vi "LBCB Conversion Unit Test.vi"() -> ()   [LabVIEW 2009]
uses:
  lib/Data Access Objects/Metadata/Actuator Point.ctl
  lib/Data Access Objects/Metadata/Cartesian Point.ctl
  lib/Data Access Objects/Metadata/Cartesian Force Vector.ctl
  lib/Data Access Objects/Metadata/LBCB Number.ctl
  lib/Data Access Objects/Metadata/LBCB Settings.ctl
  lib/Data Access Objects/Metadata/LBCB Size.ctl
  lib/Data Access Objects/Metadata/LBCB Type.ctl
  lib/Data Access Objects/Metadata/LBCB Location.ctl
  lib/Data Access Objects/Metadata/LBCB Position.ctl
  lib/Data Access Objects/Metadata/Persistant DAO Actions.ctl
  lib/Control Loop/LBCB_Conversions_Actions.ctl
panel:
  out "Filename Out":path
  in  "LBCB Position":T1={"Motion Center"=[0.0, 0.0, 0.0], "Transformation Matrix"=[[1.0, 0.0, 0.0, 0.0, 0.0, 0.0], [0.0, 1.0, 0.0, 0.0, 0.0, 0.0], [0.0, 0.0, 1.0, 0.0, 0.0, 0.0], [0.0, 0.0, 0.0, 1.0, 0.0, 0.0], [0.0, 0.0, 0.0, 0.0, 1.0, 0.0], [0.0, 0.0, 0.0, 0.0, 0.0, 1.0]]} {"Transformation Matrix" format="%#_10e"; "Motion Center" format="%#_10g"}
  in  "Save":bool
  in  "Load":bool
  in  "OM  Location":T2
  in  "Calculate":bool
  in  "LBCB Setting":T3
  in  "LBCB Number":T6
  in  "Stop":bool
  out "Forces":T7
  out "Displacements":T8
  in  "Forces Kips":T9
  in  "Displacements Inches":T9
  # "Y"
  # "(inch)"
  # "XLBCB CMD = T-1*XLBCB OM"
  # "Z"
  # "(inch)"
  # "XOM DISP = T*XLBCB DISP"
  # "(inch)"
  # "Dx"
  # "Dy"
  # "Dz"
  # "Rx"
  # "Ry"
  # "Rz"
  # "Dx"
  # "Dy"
  # "Dz"
  # "Rx"
  # "Ry"
  # "Rz"
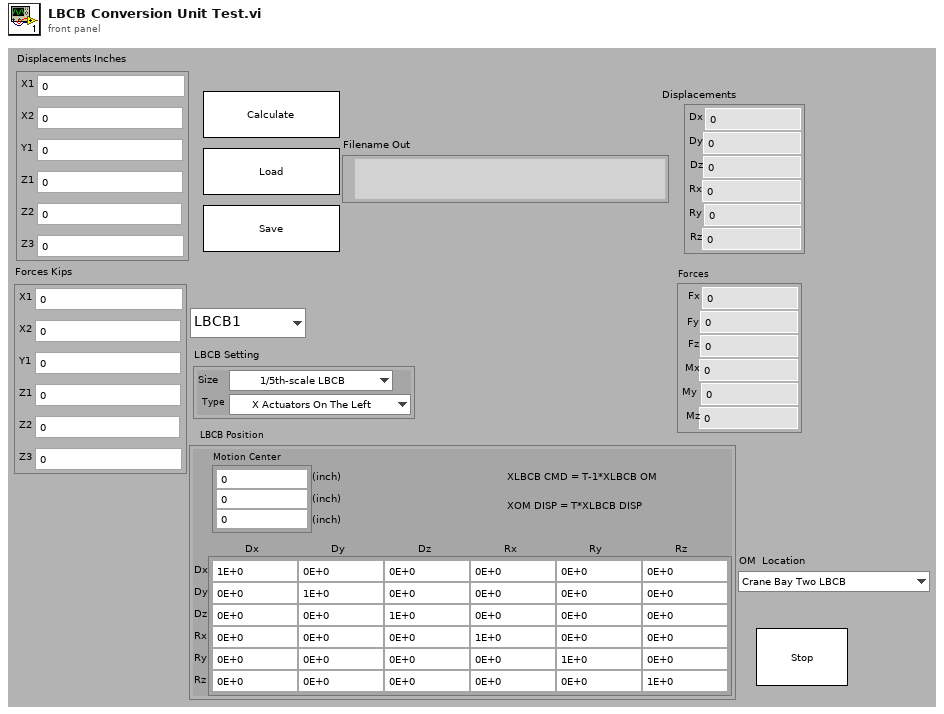
[diagram p1: front panel]
types:
  T1 = typedef "LBCB Position.ctl" = cluster{"Motion Center":dbl[], "Transformation Matrix":dbl[][]}
  T2 = typedef "LBCB Location.ctl" = enum16{"Crane Bay Two LBCB", "Crane Bay One LBCB", "5th Scale Two LBCB", "5th Scale One LBCB", "Portable LBCB"}
  T3 = typedef "LBCB Settings.ctl" = cluster{"Size":T4, "Type":T5}
  T4 = typedef "LBCB Size.ctl" = enum16{"1/5th-scale LBCB", "Full-scale LBCB", "Portable LBCB"}
  T5 = typedef "LBCB Type.ctl" = enum16{"X Actuators On The Left", "X Actuators On The Right"}
  T6 = typedef "LBCB Number.ctl" = enum16{"LBCB1", "LBCB2"}
  T7 = typedef "Cartesian Force Vector.ctl" = cluster{"Fx":dbl, "Fy":dbl, "Fz":dbl, "Mx":dbl, "My":dbl, "Mz":dbl}
  T8 = typedef "Cartesian Point.ctl" = cluster{"Dx":dbl, "Dy":dbl, "Dz":dbl, "Rx":dbl, "Ry":dbl, "Rz":dbl}
  T9 = typedef "Actuator Point.ctl" = cluster{"X1":dbl, "X2":dbl, "Y1":dbl, "Z1":dbl, "Z2":dbl, "Z3":dbl}
  T10 = typedef "Persistant DAO Actions.ctl" = enum16{"Init", "Get", "Set", "Load", "Save"}
  T11 = typedef "LBCB_Conversions_Actions.ctl" = enum16{"A2C", "C2A", "Set Log Filename", "Init"}
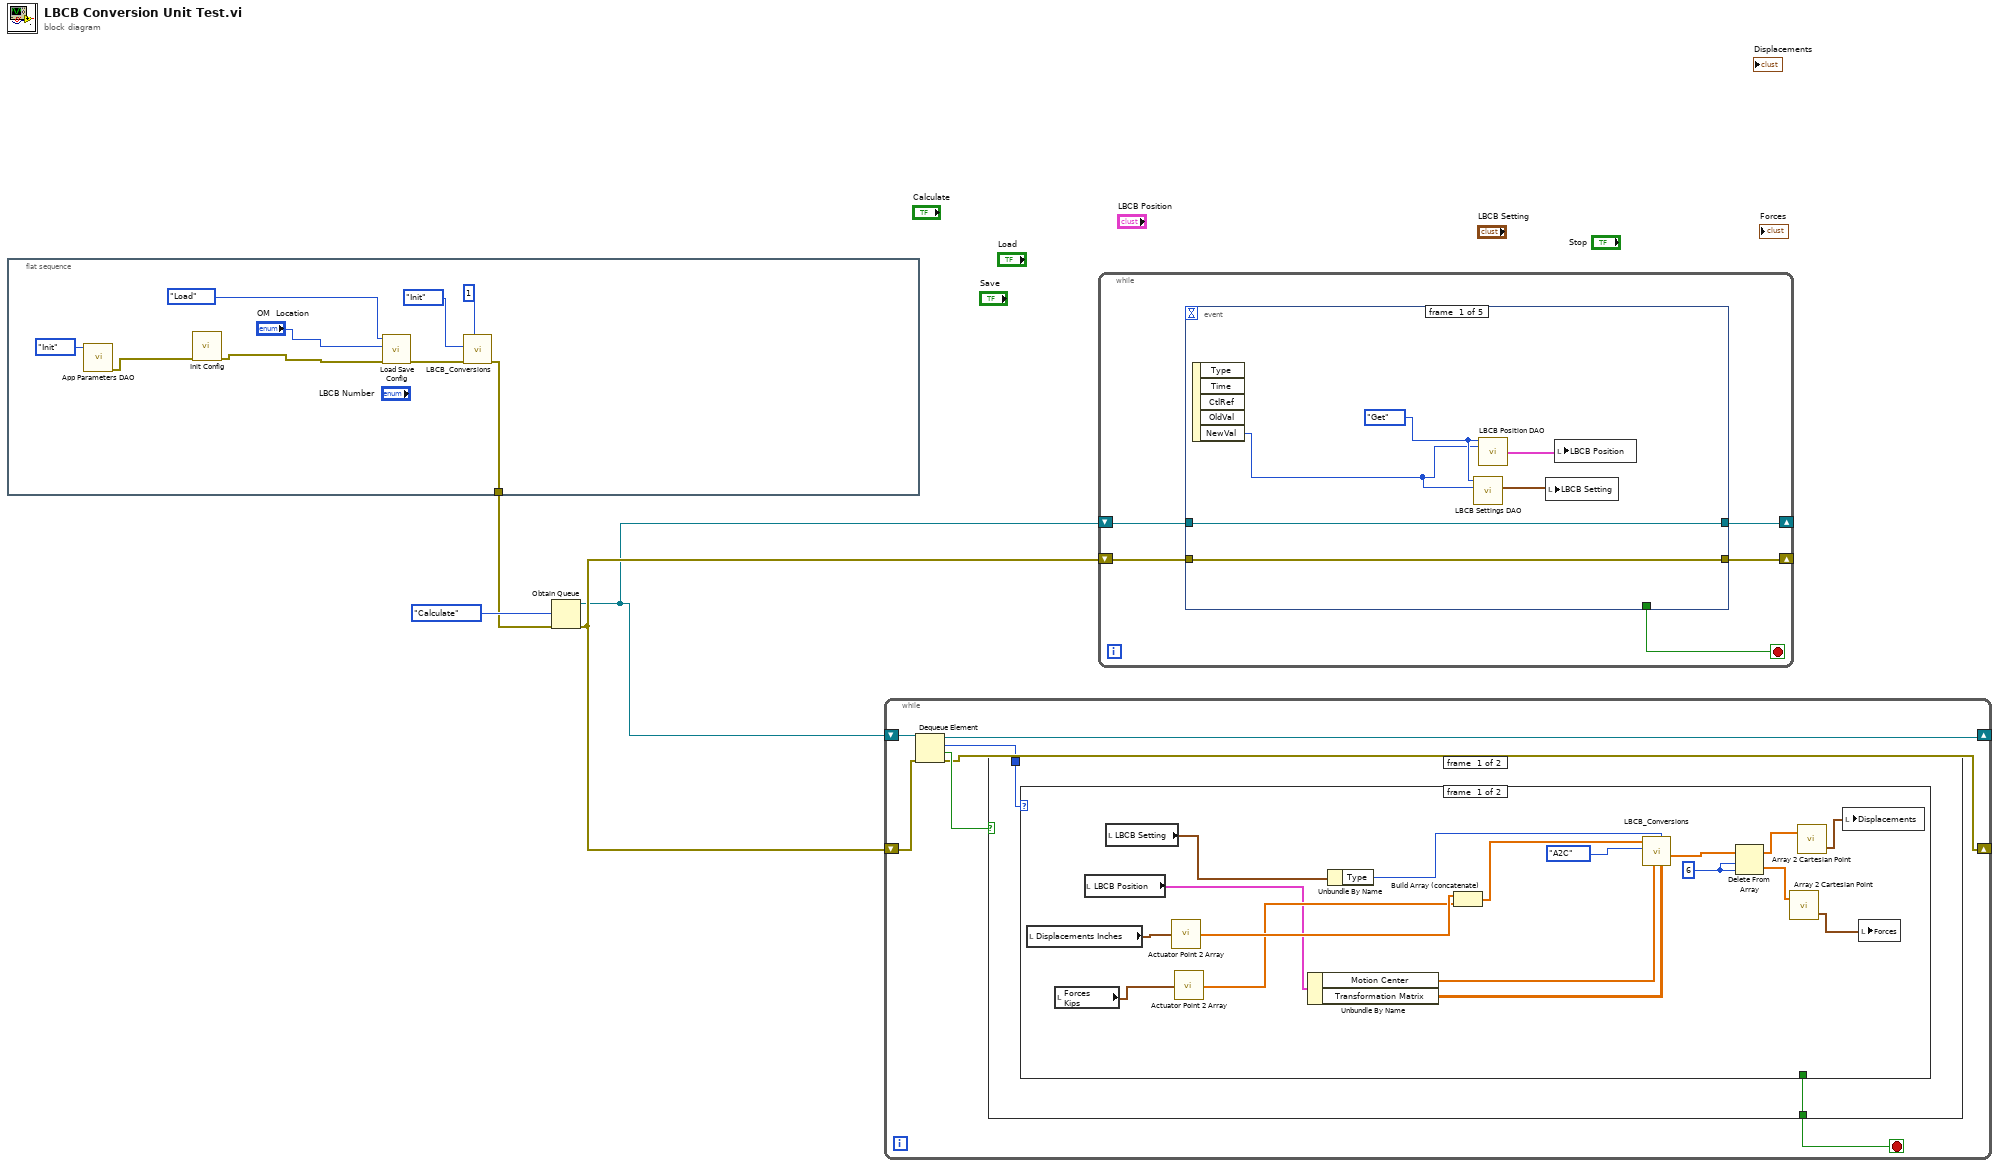
[diagram p0: block diagram]
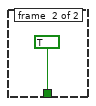
[diagram p2: hidden frame]
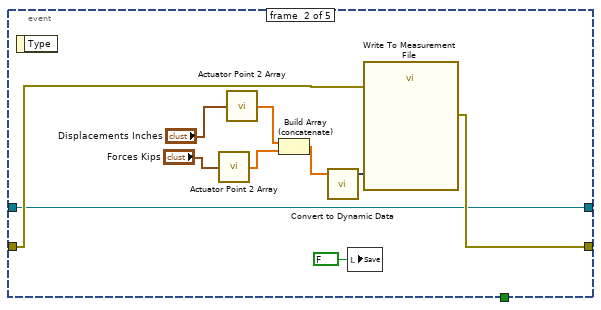
[diagram p4: hidden frame]
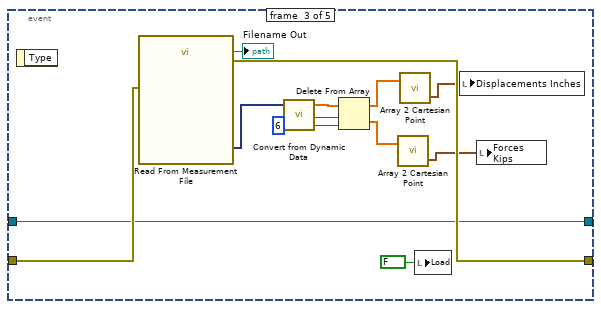
[diagram p5: hidden frame]
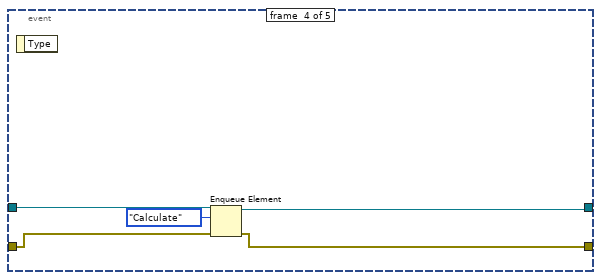
[diagram p6: hidden frame]
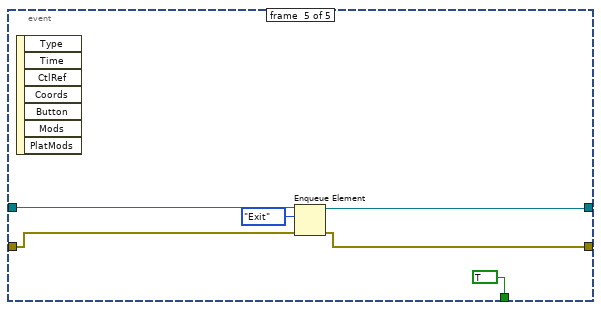
[diagram p7: hidden frame]
diagram:
  n1 = flat-sequence {
    tunnel: [w5] -> w1
    frame #0 {
      n2 = call "App Parameters DAO.vi"("Actions"=Persistant_DAO_Actions."Init") -> ("error out"=w6:errorcluster)  [unwired: 8 in, 2 out]
      n3 = call "Init Config.vi"("error in (no error)"=w6) -> ("error out"=w9:errorcluster)  [unwired: 10 in]
      n4 = call "Load Save Config.vi"("error in (no error)"=w9, "OM  Location"="OM  Location", "Actions"=Persistant_DAO_Actions."Load") -> ("error out"=w12:errorcluster)  [unwired: 8 in]
      n5 = call "LBCB_Conversions.vi"("Size"=u16 1, "error in (no error)"=w12, "Conversion Type"=LBCB_Conversions_Actions."Init") -> ("error out"=w5:errorcluster)  [unwired: 7 in, 1 out]
    }
  }
  n6 = Obtain Queue(element data type=enum16{"Calculate", "Exit"}."Calculate", error in (no error)=w1) -> (queue out=w3:refnum<queue>, error out=w4:errorcluster)  [unwired: 3 in, 1 out]
  n7 = while {
    shift-right: [w16] -> _
    shift-left: w3 -> [w19]
    shift-right: [w17] -> _
    shift-left: w4 -> [w18]
    stop <- w14 stop-if-true
    n8 = Dequeue Element(queue=w19, error in (no error)=w18) -> (queue out=w16:refnum<queue>, element=w15:enum16{"Calculate", "Exit"}, timed out?=w20:bool, error out=w17:errorcluster)  [unwired: 1 in]
    n9 = case shown="False" w20 {
      tunnel: w15 -> [w22 _]
      tunnel: [w21 _] -> w14
      frame #0 {
        n10 = case shown="\"Calculate\", Default" w22 {
          tunnel: [_ TRUE] -> w21
          frame #0 {
            w29 = 6 ("length")
            n11 = local read "Displacements Inches"() -> (w34:T9)
            n12 = local read "Forces Kips"() -> (w35:T9)
            n13 = local read "LBCB Position"() -> (w24:T1)
            n14 = local read "LBCB Setting"() -> (w23:T3)
            n15 = call "Actuator Point 2 Array.vi"("Actuator Point"=w34) -> ("Array"=w33:dbl[])
            n16 = call "Actuator Point 2 Array.vi"("Actuator Point"=w35) -> ("Array"=w32:dbl[])
            n17 = Unbundle By Name(w24) -> ("Motion Center"=w37:dbl[], "Transformation Matrix"=w36:dbl[][])
            n18 = Unbundle By Name(w23) -> ("Type"=w38:T5)
            n19 = Build Array (concatenate)(w33, w32) -> (w31:dbl[])
            n20 = call "LBCB_Conversions.vi"("Transformation Matrix"=w36, "Type"=w38, "Motion Center"=w37, "Conversion Type"=LBCB_Conversions_Actions."A2C", "Input"=w31) -> ("Output"=w30:dbl[])  [unwired: 5 in, 1 out]
            n21 = Delete From Array(array=w30, length=w29, index=w29) -> (deleted portion=w26:dbl[], array with subset deleted=w28:dbl[])
            n22 = call "Array 2 Cartesian Point.vi"("Array"=w26) -> ("Cart Disp"=w25:T8)  [unwired: 2 in]
            n23 = call "Array 2 Cartesian Point.vi"("Array"=w28) -> ("Cart Disp"=w27:T8)  [unwired: 2 in]
            n24 = local write "Displacements"(w27) -> ()
            n25 = local write "Forces"(w25) -> ()
          }
          frame #1 {
          }
        }
      }
      frame #1 {
      }
    }
  }
  n26 = while {
    shift-right: [w44] -> _
    shift-left: w3 -> [w45]
    shift-right: [w42] -> _
    shift-left: w4 -> [w43]
    stop <- w41 stop-if-true
    n27 = event shown="[2] \"Load\": Mouse Down" {
      selector: _ -> [_ _ _ _ _]
      dyn-events: _ -> [_ _ _ _ _]
      timeout: _ -> [_ _ _ _ _]
      tunnel: w45 -> [w49 w53 w70 w78 w83]
      tunnel: [w49 w53 w70 w75 w81] -> w44
      tunnel: w43 -> [w48 w55 w72 w77 w82]
      tunnel: [w48 w54 w71 w76 w80] -> w42
      tunnel: [_ _ _ _ TRUE] -> w41
      event #0 {
        w51 = Persistant_DAO_Actions."Get" ("LBCB Settings Actions")
        n28 = event-data() -> ("NewVal"=w50:T6)  [unwired: 1 in, 4 out]
        n29 = call "LBCB Settings DAO.vi"("LBCB Number"=w50, "Actions"=w51) -> ("LBCB Setting Out"=w46:T3)  [unwired: 7 in, 2 out]
        n30 = call "LBCB Position DAO.vi"("LBCB Settings Actions"=w51, "LBCB Number"=w50) -> ("LBCB Position Output"=w47:T1)  [unwired: 11 in, 2 out]
        n31 = local write "LBCB Setting"(w46) -> ()
        n32 = local write "LBCB Position"(w47) -> ()
      }
      event #1 {
        n33 = event-data() -> ()  [unwired: 1 in, 1 out]
        n34 = call "Actuator Point 2 Array.vi"("Actuator Point"="Forces Kips") -> ("Array"=w59:dbl[])
        n35 = call "Actuator Point 2 Array.vi"("Actuator Point"="Displacements Inches") -> ("Array"=w58:dbl[])
        n36 = Build Array (concatenate)(w58, w59) -> (w57:dbl[])
        n37 = call "Convert to Dynamic Data"("Array"=w57) -> ("Dynamic Data Type"=w56:dynamicdata)  [unwired: 3 in]
        n38 = local write "Save"(FALSE ("Save")) -> ()
        n39 = call "Write To Measurement File"("Signals"=w56, "error in (no error)"=w55) -> ("error out"=w54:errorcluster)  [unwired: 15 in, 2 out]
      }
      event #2 {
        w67 = 6 ("index")
        n40 = event-data() -> ()  [unwired: 1 in, 1 out]
        n41 = call "Read From Measurement File"("error in (no error)"=w72) -> ("error out"=w71:errorcluster, "Filename Out"=→"Filename Out":path, "Signals"=w69:dynamicdata)  [unwired: 5 in, 3 out]
        n42 = call "Convert from Dynamic Data"("Dynamic Data Type"=w69) -> ("Array"=w68:dbl[])  [unwired: 3 in]
        n43 = Delete From Array(array=w68, length=w67, index=w67) -> (deleted portion=w65:dbl[], array with subset deleted=w66:dbl[])
        n44 = call "Array 2 Cartesian Point.vi"("Array"=w65) -> ("Cart Disp"=w63:T8)  [unwired: 2 in]
        n45 = call "Array 2 Cartesian Point.vi"("Array"=w66) -> ("Cart Disp"=w64:T8)  [unwired: 2 in]
        n46 = local write "Load"(FALSE ("Load")) -> ()
        n47 = local write "Displacements Inches"(w64) -> ()
        n48 = local write "Forces Kips"(w63) -> ()
      }
      event #3 {
        n49 = event-data() -> ()  [unwired: 1 in, 1 out]
        n50 = Enqueue Element(queue=w78, element=enum16{"Calculate"}."Calculate", error in (no error)=w77) -> (queue out=w75:refnum<queue>, error out=w76:errorcluster)  [unwired: 1 in, 1 out]
      }
      event #4 {
        n51 = event-data() -> ()  [unwired: 1 in, 7 out]
        n52 = Enqueue Element(queue=w83, element=enum16{"Calculate", "Exit"}."Exit", error in (no error)=w82) -> (queue out=w81:refnum<queue>, error out=w80:errorcluster)  [unwired: 1 in, 1 out]
      }
    }
  }
